vi "INI read RF.vi"(8 "error in (no error)":T2, 11 "Port":string(combo)="tx") -> (0 "error out":T2, 2 "Config":T1 {"Gain" format="%#_6fdb"; "Frequency" format="%#_6pHz"}, 3 "Port out":string(combo)="tx")   [LabVIEW 2019, in "Shared.lvlib"]
uses:
  Shared.lvlib
  mmWave instrument_class/RFConfig.ctl
  System GV.vi
  <vilib>/Utility/config.llb/NI_LVConfig.lvlib
  mmWave instrument_class/mmWave instrument.lvclass
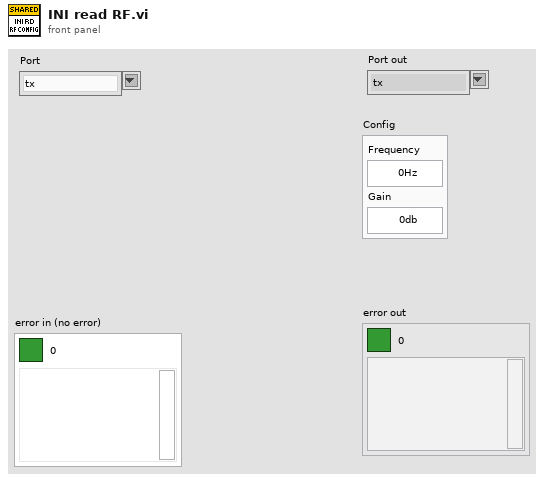
[diagram p1: front panel]
types:
  T1 = typedef "mmWave instrument.lvclass/RFConfig.ctl" = cluster{"Frequency":dbl, "Gain":dbl}
  T2 = cluster{"Boolean Round":bool, "code":i32, "source":string}
  T3 = cluster{"TX_fc":dbl, "TX_gain":dbl, "RX_fc":dbl, "RX_gain":dbl}
  T4 = typedef "NI_LVConfig.lvlib/Config Data RefNum.ctl" = refnum<k1>
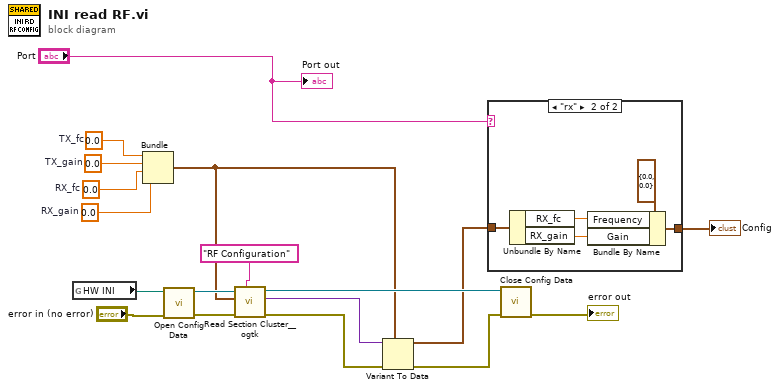
[diagram p0: block diagram]
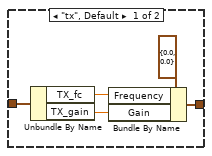
[diagram p2: hidden frame]
diagram:
  w3 = 0.0  # RX_gain
  w4 = 0.0  # RX_fc
  w5 = 0.0  # TX_gain
  w6 = 0.0  # TX_fc
  n1 = global read "System GV.vi" "HW INI"() -> (w15:path)
  n2 = Bundle("TX_fc"=w6, "TX_gain"=w5, "RX_fc"=w4, "RX_gain"=w3) -> (w10:T3)  [unwired: 1 in]
  n3 = call <vilib>:"Open Config Data.vi"("error in (no error)"="error in (no error)", "configuration file path"=w15) -> ("error out"=w16:errorcluster, "refnum"=w18:T4)  [unwired: 7 in, 1 out]
  n4 = call <userlib>:"Read Section Cluster__ogtk.vi"("section (optional)"="RF Configuration", "error in (no error)"=w16, "Section Formatted Cluster Type"=w10, "refnum"=w18) -> ("error out"=w12:errorcluster, "Section Formatted Cluster"=w13:variant, "dup refnum"=w17:T4)  [unwired: 3 in, 2 out]
  n5 = Variant To Data(error in=w12, type=w10, Variant=w13) -> (data=w9:T3, error out=w11:errorcluster)
  n6 = case shown="\"rx\"" "Port" {
    tunnel: w9 -> [w23 w28]
    tunnel: [w19 w24] -> w1
    frame "tx", Default {
      n7 = Unbundle By Name(w23) -> ("TX_fc"=w20:dbl, "TX_gain"=w21:dbl)
      n8 = Bundle By Name(cluster=T1 {"Frequency"=0.0, "Gain"=0.0} ("Config 2"), "Frequency"=w20, "Gain"=w21) -> (w19:T1)
    }
    frame "rx" {
      n9 = Unbundle By Name(w28) -> ("RX_fc"=w25:dbl, "RX_gain"=w26:dbl)
      n10 = Bundle By Name(cluster=T1 {"Frequency"=0.0, "Gain"=0.0} ("Config 2"), "Frequency"=w25, "Gain"=w26) -> (w24:T1)
    }
  }
  "Config" <- w1
  n11 = call <vilib>:"Close Config Data.vi"("error in (no error)"=w11, "refnum"=w17) -> ("error out"=→"error out":errorcluster)  [unwired: 8 in, 1 out]
  "Port out" <- "Port"
